vi "MultiChannel Write.vi"(8 "错误输入":cluster{"状态":bool, "代码":i32, "源":string}, 10 "数据至记录":dbl[][](array[numeric]), 11 "文件引用句柄输入":refnum<file>) -> (0 "错误输出":cluster{"状态":bool, "代码":i32, "源":string}, 3 "文件引用句柄输出":refnum<file>)   [LabVIEW 2012]
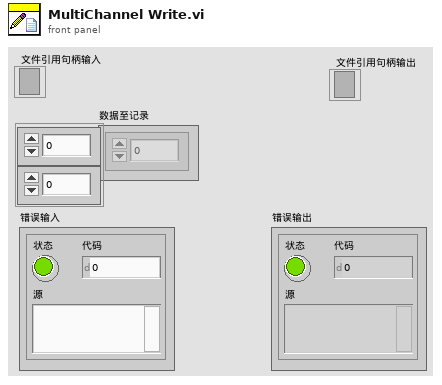
[diagram p1: front panel]
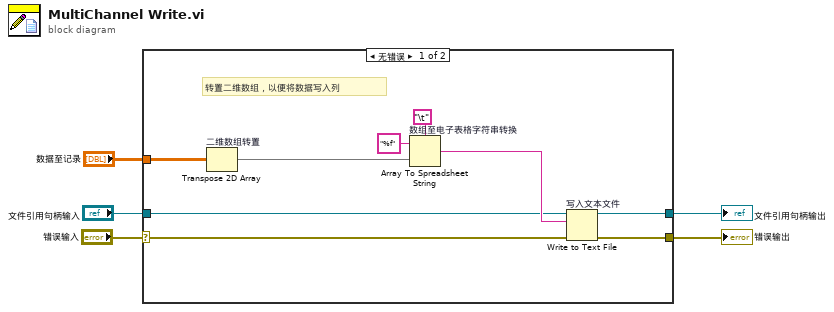
[diagram p0: block diagram]
diagram:
  n1 = case shown="无错误" "错误输入" {
    selector: "错误输入" -> [w14 w16]
    tunnel: "文件引用句柄输入" -> [w7 w15]
    tunnel: [w6 w15] -> w3
    tunnel: [w13 w16] -> w2
    tunnel: "数据至记录" -> [w9 _]
    frame No Error {
      # "转置二维数组，以便将数据写入列"
      n2 = Transpose 2D Array "二维数组转置"(2D array=w9) -> (transposed array=w8:dbl[][])
      n3 = Array To Spreadsheet String "数组至电子表格字符串转换"(delimiter (Tab)="\t" ("制表符常量"), array=w8, 3:"%f" ("格式字符串")) -> (spreadsheet string=w12:string)
      n4 = Write to Text File "写入文本文件"(file (use dialog)=w7, text=w12, error in=w14) -> (refnum out=w6:refnum<file>, error out=w13:errorcluster)  [unwired: 1 in, 1 out]
    }
    frame Error {
    }
  }
  "错误输出" <- w2
  "文件引用句柄输出" <- w3
